vi "Read Status Byte Query.vi"(0 "VISA resource name":refnum<visa-resource-name>, 11 "error in (no error)":errorcluster) -> (4 "VISA resource name out":refnum<visa-resource-name>, 6 "Status Byte Register":T1, 15 "error out":errorcluster)   [LabVIEW 2014, in "eec 6700.lvlib"]
doc: "Queries the <B>Status Byte</B>. Returns the decimal value of the binary-weighted sum of bits.\n\nEach bit represents a status in the instrument.\n\nEx : When Test passes, BIT 0 is set High giving status \"ALL PASS\"\n\nBIT 0 ,01H,(1) All PASS\nBIT 1 ,02H,(2) FAIL\nBIT 2, 04H,(4) ABORT\nBIT 3, 08H,(8) Process\nBIT 4, 10H,(16) Message Available\nBIT 5, 20H,(32) Standard Event (ESB)\nBIT 6, 40H,(64) Request Service (MSS)\nBIT 7, 80H,(128) Prompt"
uses:
  <instrlib>/eec 6700/eec 6700.lvlib
panel:
  # "BIT 0 ,01H,(1)   All PASS\nBIT 1 ,02H,(2)   FAIL\nBIT 2, 04H,(4)   ABORT\nBIT 3, 08H,(8)   Process\nBIT 4, 10H,(16)  Message Available\nBIT 5, 20H,(32)  Standard Event  (ESB)\nBIT 6, 40H,(64)  Request Service (MSS)\nBIT 7, 80H,(128) Prompt"
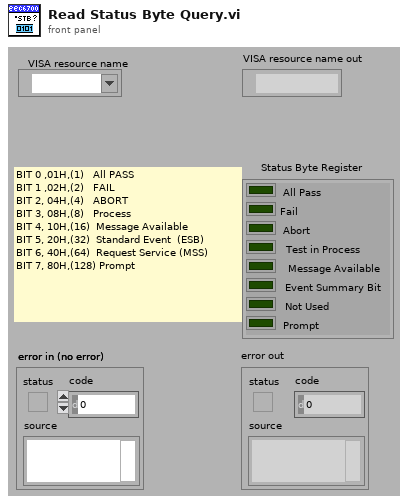
[diagram p1: front panel]
types:
  T1 = cluster{"All Pass":bool, "Fail":bool, "Abort":bool, "Test in Process":bool, "Message Available":bool, "Event Summary Bit":bool, "Not Used":bool, "Prompt":bool}
  T2 = cluster{"Boolean array[0]":bool, "Boolean array[1]":bool, "Boolean array[2]":bool, "Boolean array[3]":bool, "Boolean array[4]":bool, "Boolean array[5]":bool, "Boolean array[6]":bool, "Boolean array[7]":bool}
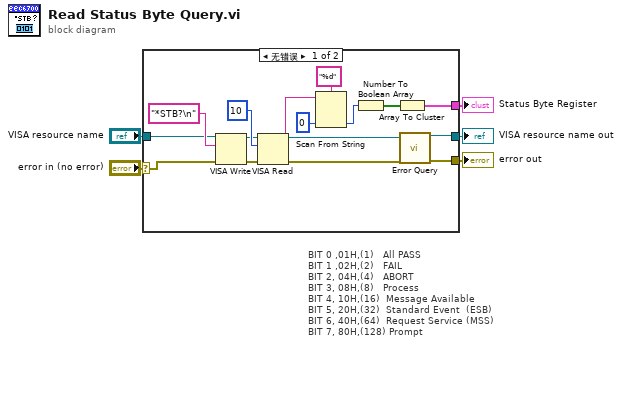
[diagram p0: block diagram]
diagram:
  # "BIT 0 ,01H,(1)   All PASS\nBIT 1 ,02H,(2)   FAIL\nBIT 2, 04H,(4)   ABORT\nBIT 3, 08H,(8)   Process\nBIT 4, 10H,(16)  Message Available\nBIT 5, 20H,(32)  Standard Event  (ESB)\nBIT 6, 40H,(64)  Request Service (MSS)\nBIT 7, 80H,(128) Prompt"
  n1 = case shown="无错误" "error in (no error)" {
    selector: "error in (no error)" -> [w10 w22]
    tunnel: [w21 _] -> w5
    tunnel: "VISA resource name" -> [w9 w23]
    tunnel: [w20 w23] -> w3
    tunnel: [w19 w22] -> w2
    frame No Error {
      n2 = VISA Write(VISA resource name=w9, write buffer="*STB?\n" ("Command to Send (empty)"), error in (no error)=w10) -> (VISA resource name out=w15:refnum<visa-resource-name>, error out=w14:errorcluster)  [unwired: 1 out]
      n3 = VISA Read(VISA resource name=w15, byte count=u32 10, error in (no error)=w14) -> (VISA resource name out=w8:refnum<visa-resource-name>, read buffer=w17:string, error out=w7:errorcluster)  [unwired: 1 out]
      n4 = Scan From String(format string="%d" ("Format String"), input string=w17, default 1=u8 0 ("default value 1")) -> (output 1=w6:u8)  [unwired: 2 in, 3 out]
      n5 = Number To Boolean Array(number=w6) -> (Boolean array=w18:bool[])
      n6 = Array To Cluster(array=w18) -> (cluster=w21:T2)
      n7 = call <instrlib>:"Error Query.vi"("VISA resource name"=w8, "error in (no error)"=w7) -> ("VISA resource name out"=w20:refnum<visa-resource-name>, "error out"=w19:errorcluster)  [unwired: 10 in, 2 out]
    }
    frame Error {
    }
  }
  "Status Byte Register" <- w5
  "VISA resource name out" <- w3
  "error out" <- w2
